vi "test.vi"() -> ()   [LabVIEW 2018]
uses:
  CubeLogger/File.ctl
  CubeLogger/Dataset.ctl
  CubeLogger/CubeLogger.lvclass
panel:
  in  "ScanSteps":i32=10
  in  "File":T1={"Name"="try", "Folder"=path "D:/temp", "Description"="..."}
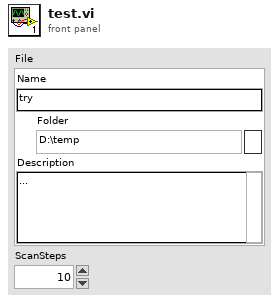
[diagram p1: front panel]
types:
  T1 = typedef "CubeLogger.lvclass/File.ctl" = cluster{"Name":string, "Folder":path, "Description":string}
  T2 = typedef "CubeLogger.lvclass/Dataset.ctl" = cluster{"name":string, "path":string, "size":i32[], "type":enum16{"single", "double", "uint8", "uint16", "uint32", "uint64", "int8", "int16", "int32", "int64"}, "mfmt":string}
  T3 = cluster{"File":T1, "CubeLogger.lvclass:Dataset":T2}
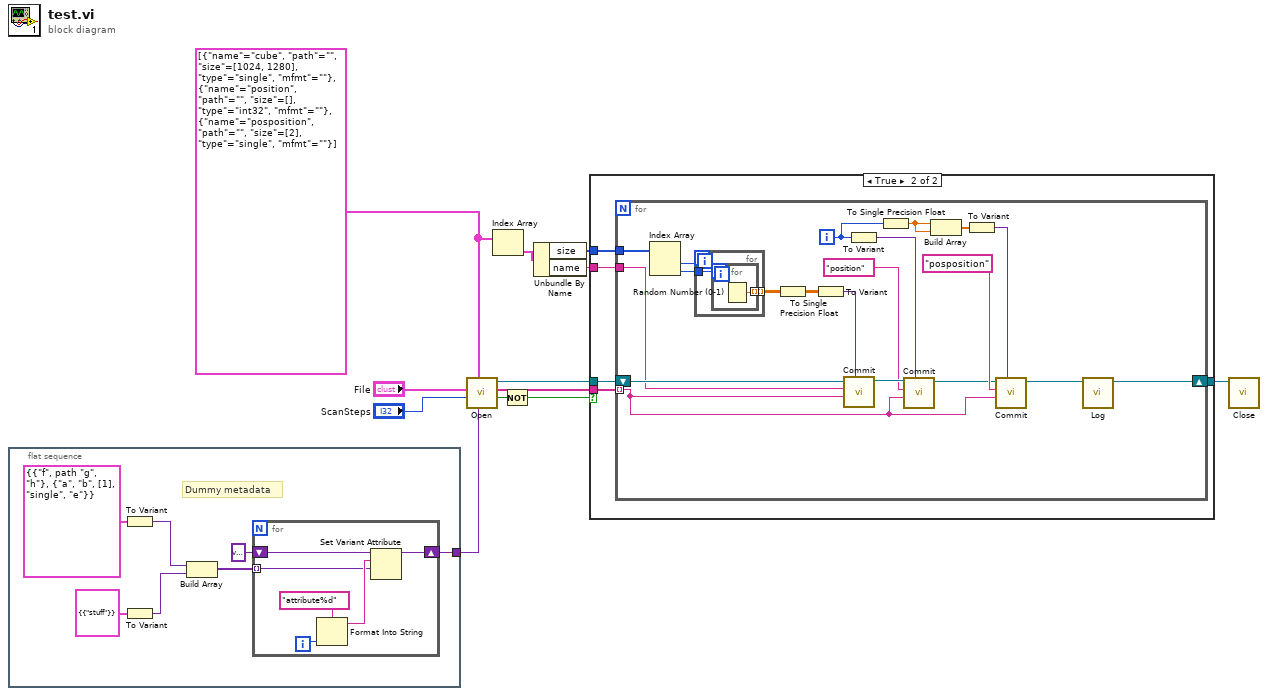
[diagram p0: block diagram]
diagram:
  w5 = T2[] [{"name"="cube", "path"="", "size"=[1024, 1280], "type"=enum."single", "mfmt"=""}, {"name"="position", "path"="", "size"=[], "type"=enum."int32", "mfmt"=""}, {"name"="posposition", "path"="", "size"=[2], "type"=enum."single", "mfmt"=""}] ("Dataset[]")
  n1 = flat-sequence {
    tunnel: [w19] -> w12
    frame #0 {
      # "Dummy metadata"
      n2 = To Variant(anything=T3 {"File"={"Name"="f", "Folder"=path "g", "Description"="h"}, "CubeLogger.lvclass:Dataset"={"name"="a", "path"="b", "size"=[1], "type"=enum."single", "mfmt"="e"}}) -> (Variant=w14:variant)
      n3 = To Variant(anything=cluster{cluster{"meta":string}} {{"meta"="stuff"}}) -> (Variant=w13:variant)
      n4 = Build Array(w14, w13) -> (w17:variant[])
      n5 = for {
        shift-right: [w23] -> w19
        shift-left: variant -> [w22]
        tunnel: w17 -> [w20] mode=indexing
        i -> [w25]
        n6 = Format Into String(format string="attribute%d", w25) -> (resulting string=w21:string)  [unwired: 2 in, 1 out]
        n7 = Set Variant Attribute(Variant=w22, name=w21, value=w20) -> (Variant out=w23:variant)  [unwired: 1 in, 2 out]
      }
    }
  }
  n8 = call "Open.vi"("Metadata"=w12, "Dataset[]"=w5, "ScanSteps"="ScanSteps", "File"="File") -> ("Canceled?"=w9:bool, "UUID[]"=w6:string[], "CubeLogger out"=w7:refnum<class "CubeLogger.lvclass">)  [unwired: 4 in, 1 out]
  n9 = Index Array(array=w5) -> (element=w4:T2)  [unwired: 1 in]
  n10 = Not(x=w9) -> (.not. x?=w8:bool)
  n11 = Unbundle By Name(w4) -> ("size"=w3:i32[], "name"=w1:string)
  n12 = case shown="True" w8 {
    tunnel: w7 -> [w26 w29]
    tunnel: w6 -> [_ w31]
    tunnel: w3 -> [_ w30]
    tunnel: [w26 w28] -> w2
    tunnel: w1 -> [_ w27]
    frame False {
    }
    frame True {
      n13 = for {
        tunnel: w31 -> [w38] mode=indexing
        tunnel: w30 -> [w51]
        shift-right: [w46] -> w28
        shift-left: w29 -> [w47]
        tunnel: w27 -> [w40]
        i -> [w37]
        n14 = Index Array(array=w51) -> (element #1=w50:i32, element #2=w49:i32)  [unwired: 2 in]
        n15 = for {
          N: w50 -> [_]
          tunnel: w49 -> [w53]
          tunnel: [w52] -> w48 mode=indexing
          n16 = for {
            N: w53 -> [_]
            tunnel: [w54] -> w52 mode=indexing
            n17 = Random Number (0-1)() -> (number: 0 to 1=w54:dbl)
          }
        }
        n18 = To Single Precision Float(number=w48) -> (single precision float=w45:sgl[][])
        n19 = To Variant(anything=w45) -> (Variant=w44:variant)
        n20 = call "Commit.vi"("Data"=w44, "UUID"=w38, "Dataset"=w40, "CubeLogger in"=w47) -> ("CubeLogger out"=w43:refnum<class "CubeLogger.lvclass">)  [unwired: 4 in, 3 out]
        n21 = To Variant(anything=w37) -> (Variant=w42:variant)
        n22 = To Single Precision Float(number=w37) -> (single precision float=w36:sgl)
        n23 = call "Commit.vi"("Data"=w42, "UUID"=w38, "Dataset"="position", "CubeLogger in"=w43) -> ("CubeLogger out"=w33:refnum<class "CubeLogger.lvclass">)  [unwired: 4 in, 3 out]
        n24 = Build Array(w36, w36) -> (w35:sgl[])
        n25 = To Variant(anything=w35) -> (Variant=w34:variant)
        n26 = call "Commit.vi"("Data"=w34, "UUID"=w38, "Dataset"="posposition", "CubeLogger in"=w33) -> ("CubeLogger out"=w32:refnum<class "CubeLogger.lvclass">)  [unwired: 4 in, 3 out]
        n27 = call "Log.vi"("CubeLogger in"=w32) -> ("CubeLogger out"=w46:refnum<class "CubeLogger.lvclass">)  [unwired: 5 in, 5 out]
      }
    }
  }
  n28 = call "Close.vi"("CubeLogger in"=w2) -> ()  [unwired: 8 in, 3 out]
